vi "Check Status.vi"(8 "error in (no error)":errorcluster, 11 "Microwave in":refnum<class "Microwave.lvclass">) -> (0 "error out":errorcluster, 1 "Status":string, 2 "Ready?":bool, 3 "Microwave out":refnum<class "Microwave.lvclass">)   [LabVIEW 2023, in "Microwave.lvclass"]
doc: "(Dynamic) Check if the instrument is powered on and update its member data with the instrument's current status. Optionally return a text status message."
uses:
  Microwave.lvclass
  Microwave.lvclass/Microwave.ctl
  Utility Classes/Scannable/Scannable.lvclass
  Agilent PSG MXG Series/Agilent PSG MXG Series.lvlib
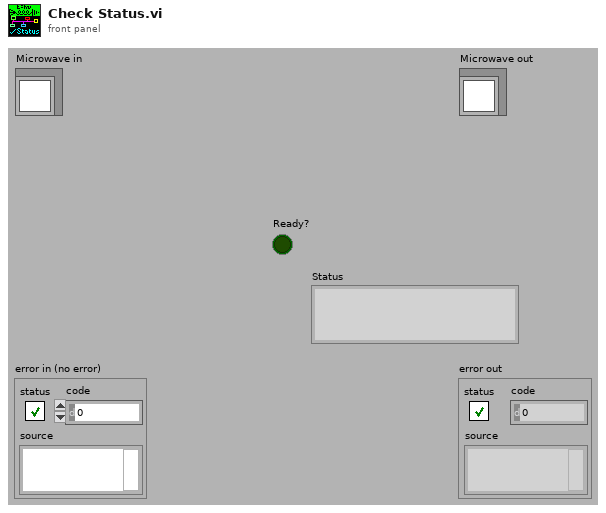
[diagram p1: front panel]
types:
  T1 = enum16{"CW", "Fixed", "Stepped Sweep", "List Sweep"}
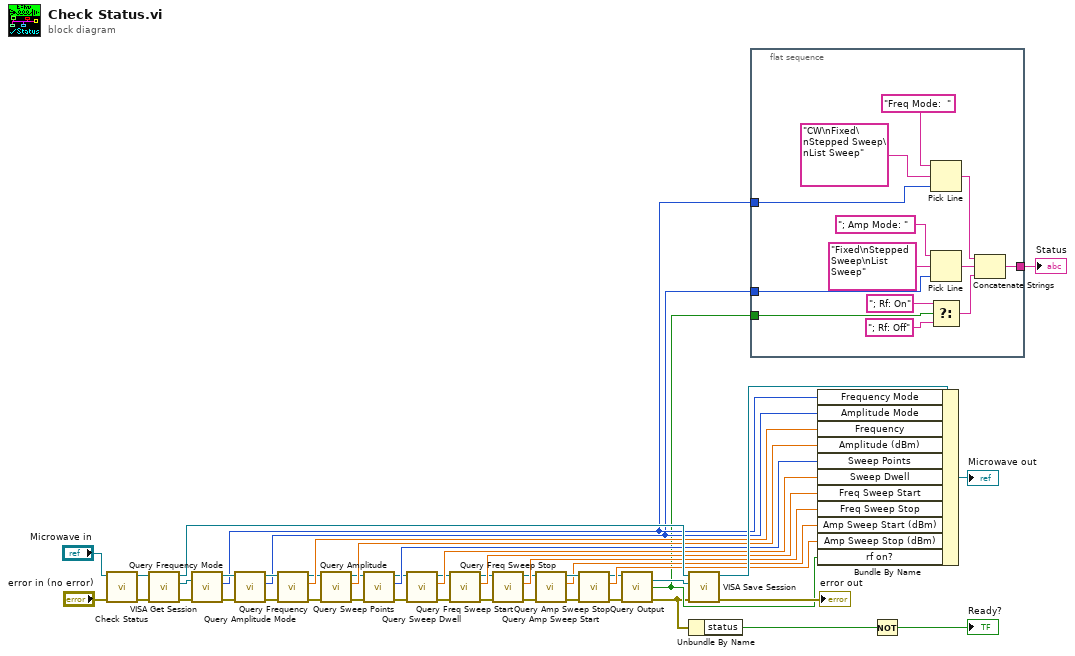
[diagram p0: block diagram]
diagram:
  n1 = call-parent "Check Status.vi"("error in (no error)"="error in (no error)", "Instrument in"="Microwave in") -> ("error out"=w41:errorcluster, "Instrument out"=w42:refnum<class "Microwave.lvclass">)  [unwired: 8 out]
  n2 = call-dynamic "VISA Get Session.vi"("error in (no error)"=w41, "Instrument.lvclass in"=w42) -> ("error out"=w4:errorcluster, "VISA Resource Name"=w5:refnum<visa-resource-name>, "Instrument.lvclass out"=w43:refnum<class "Microwave.lvclass">)  [unwired: 7 out]
  n3 = call "Query Frequency Mode.vi"("error in (no error)"=w4, "VISA resource name"=w5) -> ("error out"=w3:errorcluster, "Frequency Mode"=w8:T1, "VISA resource name out"=w37:refnum<visa-resource-name>)  [unwired: 7 out]
  n4 = call "Query Amplitude Mode.vi"("error in (no error)"=w3, "VISA resource name"=w37) -> ("error out"=w35:errorcluster, "Amplitude Mode"=w7:enum16{"Fixed", "Stepped Sweep", "List Sweep"}, "VISA resource name out"=w36:refnum<visa-resource-name>)  [unwired: 7 out]
  n5 = call "Query Frequency.vi"("error in (no error)"=w35, "VISA resource name"=w36) -> ("error out"=w32:errorcluster, "Frequency"=w34:dbl[unit], "VISA resource name out"=w33:refnum<visa-resource-name>)  [unwired: 7 out]
  n6 = call "Query Amplitude.vi"("error in (no error)"=w32, "VISA resource name"=w33) -> ("error out"=w29:errorcluster, "Amplitude (dBm)"=w31:dbl, "VISA resource name out"=w30:refnum<visa-resource-name>)  [unwired: 7 out]
  n7 = call "Query Sweep Points.vi"("error in (no error)"=w29, "VISA resource name"=w30) -> ("error out"=w26:errorcluster, "Number of Sweep Points"=w28:i32, "VISA resource name out"=w27:refnum<visa-resource-name>)  [unwired: 7 out]
  n8 = call "Query Sweep Dwell.vi"("error in (no error)"=w26, "VISA resource name"=w27) -> ("error out"=w23:errorcluster, "Sweep Dwell Time"=w25:dbl[unit], "VISA resource name out"=w24:refnum<visa-resource-name>)  [unwired: 7 out]
  n9 = call "Query Freq Sweep Start.vi"("error in (no error)"=w23, "VISA resource name"=w24) -> ("error out"=w20:errorcluster, "Frequency Sweep Start"=w22:dbl[unit], "VISA resource name out"=w21:refnum<visa-resource-name>)  [unwired: 7 out]
  n10 = call "Query Freq Sweep Stop.vi"("error in (no error)"=w20, "VISA resource name"=w21) -> ("error out"=w15:errorcluster, "Frequency Sweep Stop"=w19:dbl[unit], "VISA resource name out"=w16:refnum<visa-resource-name>)  [unwired: 7 out]
  n11 = call "Query Amp Sweep Start.vi"("error in (no error)"=w15, "VISA resource name"=w16) -> ("error out"=w17:errorcluster, "Amplitude Sweep Start (dBm)"=w14:dbl, "VISA resource name out"=w18:refnum<visa-resource-name>)  [unwired: 7 out]
  n12 = call "Query Amp Sweep Stop.vi"("error in (no error)"=w17, "VISA resource name"=w18) -> ("error out"=w10:errorcluster, "Amplitude Sweep Stop (dBm)"=w13:dbl, "VISA resource name out"=w12:refnum<visa-resource-name>)  [unwired: 7 out]
  n13 = call "Query Output.vi"("error in (no error)"=w10, "VISA resource name"=w12) -> ("error out"=w1:errorcluster, "Output On?"=w6:bool, "VISA resource name out"=w11:refnum<visa-resource-name>)  [unwired: 7 out]
  n14 = call-dynamic "VISA Save Session.vi"("error in (no error)"=w1, "VISA Resource Name"=w11, "Instrument.lvclass in"=w43) -> ("error out"=→"error out":errorcluster, "Instrument.lvclass out"=w39:refnum<class "Microwave.lvclass">)  [unwired: 7 out]
  n15 = Unbundle By Name(w1) -> ("status"=w40:bool)
  n16 = flat-sequence {
    tunnel: [w57] -> w9
    tunnel: w8 -> [w53]
    tunnel: w7 -> [w52]
    tunnel: w6 -> [w48]
    frame #0 {
      n17 = Pick Line(string ("")="Freq Mode:  ", multi-line string="CW\nFixed\nStepped Sweep\nList Sweep", line index=w53) -> (output string=w58:string)
      n18 = Pick Line(string ("")="; Amp Mode: ", multi-line string="Fixed\nStepped Sweep\nList Sweep", line index=w52) -> (output string=w51:string)
      n19 = Select(t="; Rf: On" ("string (\"\")"), s=w48, f="; Rf: Off" ("string (\"\")")) -> (s? t:f=w47:string)
      n20 = Concatenate Strings(w58, w51, w47) -> (w57:string)
    }
  }
  n21 = Bundle By Name(cluster=w39, "Frequency Mode"=w8, "Amplitude Mode"=w7, "Frequency"=w34, "Amplitude (dBm)"=w31, "Sweep Points"=w28, "Sweep Dwell"=w25, "Freq Sweep Start"=w22, "Freq Sweep Stop"=w19, "Amp Sweep Start (dBm)"=w14, "Amp Sweep Stop (dBm)"=w13, "rf on?"=w6) -> (→"Microwave out":refnum<class "Microwave.lvclass">)
  n22 = Not(x=w40) -> (.not. x?=→"Ready?":bool)
  "Status" <- w9
